vi "test_SomeSessionsRegistered_CallCreateSessionsWithAttachAndClose_InitializeCalledWithProperBehavior.vi"(8 "error in":errorcluster) -> (0 "error out":errorcluster, 2 "result":string, 3 "pass":bool)   [LabVIEW 2020, in "MeasurementServerTests.lvlib"]
uses:
  MeasurementServerTests.lvlib
  Runtime/MeasurementLink Session Management/Session Reservation/Initialize and Close Session Behavior.ctl
  Runtime/MeasurementLink Session Management/Session Reservation/Session Reservation.lvclass
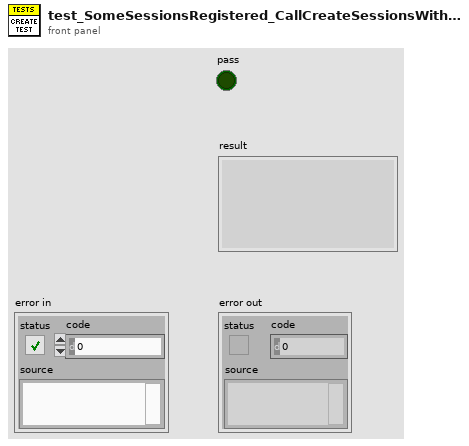
[diagram p1: front panel]
types:
  T1 = typedef "MeasurementLink Session Management.lvlib/Session Reservation.lvclass/Initialize and Close Session Behavior.ctl" = enum16{"Auto", "Initialize and Close", "Attach and Detach", "Initialize and Detach", "Attach and Close"}
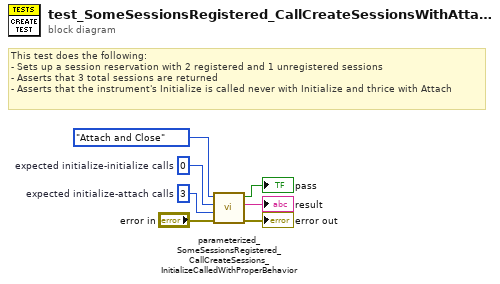
[diagram p0: block diagram]
diagram:
  w3 = u32 3  # expected initialize-attach calls
  w2 = u32 0  # expected initialize-initialize calls
  # "This test does the following:\n- Sets up a session reservation with 2 registered and 1 unregistered sessions\n- Asserts that 3 total sessions are returned\n- Asserts that the instrument's Initialize is called never with Initialize and thrice with Attach"
  n1 = call "parameterized_SomeSessionsRegistered_CallCreateSessions_InitializeCalledWithProperBehavior.vi"("error in"="error in", "expected initialize-attach calls"=w3, "expected initialize-initialize calls"=w2, "initialize and close session behavior"=Initialize_and_Close_Session_Behavior."Attach and Close") -> ("error out"=→"error out":errorcluster, "result"=→"result":string, "pass"=→"pass":bool)  [unwired: 5 in]
